vi "主副屏通信slave.vi"() -> ()   [LabVIEW 2016, in "斯坦道多参数.lvlib"]
uses:
  <vilib>/NI/Modbus Library/Network Protocol/Network Slave/TCP/Connection.ctl
  <vilib>/NI/Modbus Library/API/Wrapper/Create TCP Slave.vi
  <vilib>/NI/Modbus Library/API/slave/Modbus Slave.lvclass
  <vilib>/NI/Modbus Library/API/Wrapper/API Main.lvlib
  <vilib>/NI/Modbus Library/Network Protocol/Network Slave/TCP/TCP Slave.lvclass
panel:
  out "TCP Connection List":T1[](array[typedef])
  out "TCP Connection Count":u32
  in  "停止":bool
  out "read values":u16[](array[numeric])
  in  "write values":u16[](array[numeric])
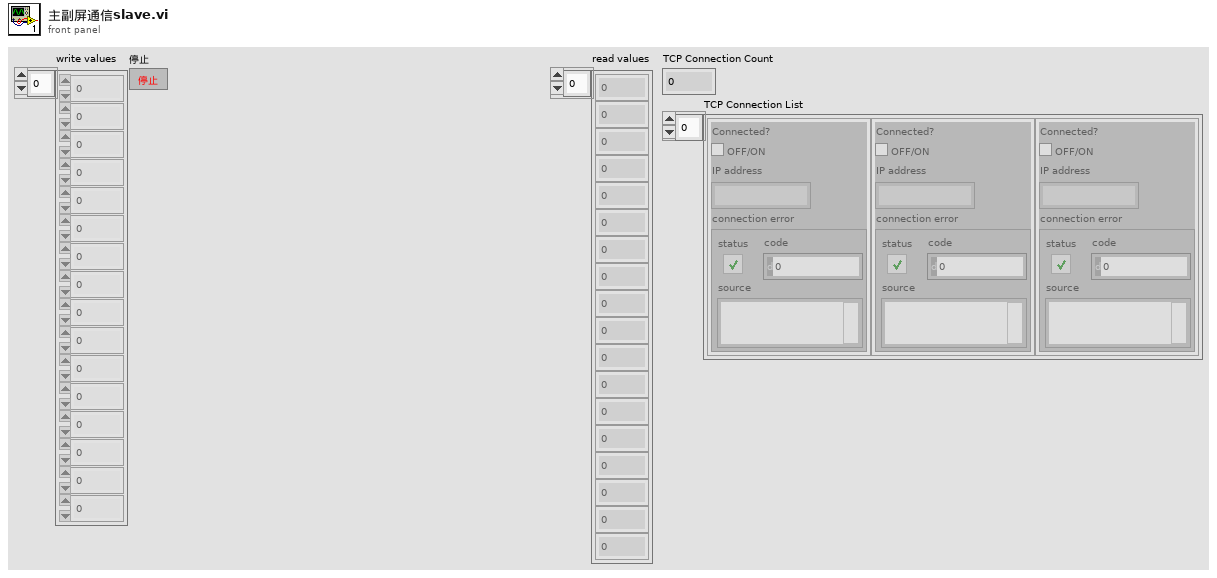
[diagram p1: front panel]
types:
  T1 = typedef "TCP Slave.lvclass/Connection.ctl" = cluster{"Connected?":bool, "IP address":string, "connection error":errorcluster}
  T2 = cluster{"数据保存间隔":dbl, "保存组数":dbl, "水温标样值":dbl, "pH标样值":dbl, "溶解氧标样值":dbl, "电导率标样值":dbl, "浊度标样值":dbl, "pH启用":bool, "溶解氧启用":bool, "电导率启用":bool, "浊度启用":bool}
  T3 = cluster{"数据保存间隔":dbl, "水温标样值":dbl, "pH标样值":dbl, "溶解氧标样值":dbl, "电导率标样值":dbl, "浊度标样值":dbl}
  T4 = cluster{"ph":bool, "DO":bool, "Cond":bool, "Turb":bool, "叶绿素a":bool, "藻密度":bool, "ORP":bool, "COD":bool}
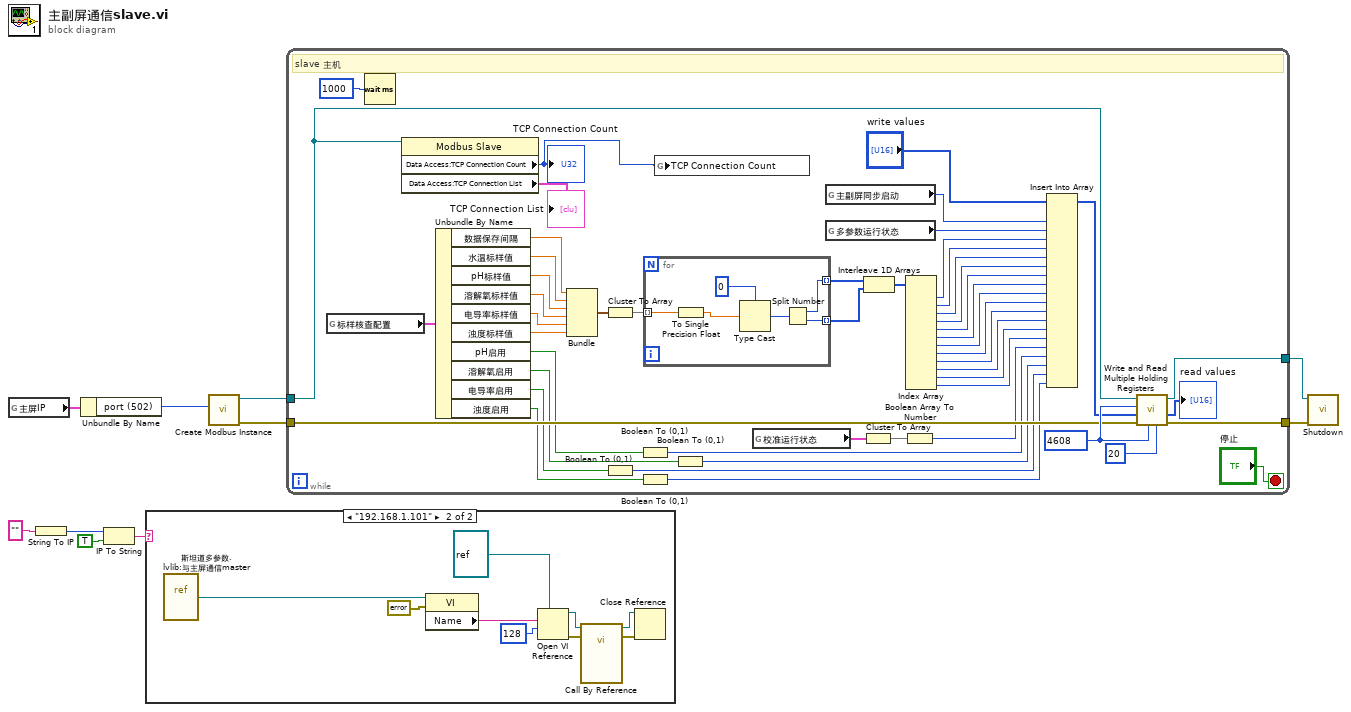
[diagram p0: block diagram]
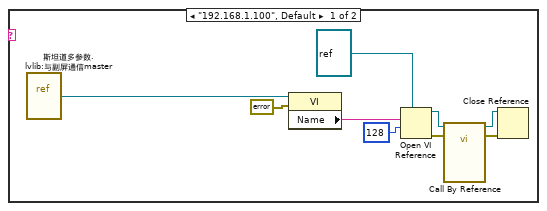
[diagram p2: hidden frame]
diagram:
  n1 = global read "多参数全局变量.vi" "主屏IP"() -> (w6:cluster{"address":string, "port (502)":u16})
  n2 = String To IP(1:"" ("名称")) -> (0:w4:u32)
  n3 = Unbundle By Name(w6) -> ("port (502)"=w5:u16)
  n4 = IP To String(1:TRUE ("句点符号？(F)"), 2:w4) -> (0:w1:string)
  n5 = case shown="\"192.168.1.101\"" w1 {
    frame "192.168.1.100", Default {
      n6 = vi-ref "斯坦道多参数.lvlib:与副屏通信master.vi"() -> (w11:refnum<vi>)
      n7 = property class="VI"(reference=w11, error in=errorcluster {"status"=FALSE, "code"=0, "source"=""} ("错误输出")) -> ("Name"=w12:string)  [unwired: 2 out]
      n8 = Open VI Reference(type specifier VI Refnum (for type only)=refnum<vi> refnum, vi path=w12, options=128 ("选项")) -> (vi reference=w14:refnum<vi>, error out=w16:errorcluster)  [unwired: 3 in]
      n9 = call-by-ref "?"(reference=w14, error in=w16) -> (reference out=w18:refnum<vi>, error out=w17:errorcluster)  [unwired: 12 in]
      n10 = Close Reference(reference=w18, error in (no error)=w17) -> ()  [unwired: 1 out]
    }
    frame "192.168.1.101" {
      n11 = vi-ref "斯坦道多参数.lvlib:与主屏通信master.vi"() -> (w20:refnum<vi>)
      n12 = property class="VI"(reference=w20, error in=errorcluster {"status"=FALSE, "code"=0, "source"=""} ("错误输出")) -> ("Name"=w21:string)  [unwired: 2 out]
      n13 = Open VI Reference(type specifier VI Refnum (for type only)=refnum<vi> refnum, vi path=w21, options=128 ("选项")) -> (vi reference=w23:refnum<vi>, error out=w25:errorcluster)  [unwired: 3 in]
      n14 = call-by-ref "?"(reference=w23, error in=w25) -> (reference out=w27:refnum<vi>, error out=w26:errorcluster)  [unwired: 12 in]
      n15 = Close Reference(reference=w27, error in (no error)=w26) -> ()  [unwired: 1 out]
    }
  }
  n16 = call-poly <vilib>:"Create Modbus Instance.vi"("port (502)"=w5) -> ("error out"=w7:errorcluster, "TCP slave instance"=w10:refnum<class "Modbus Slave.lvclass">)  [unwired: 9 in]
  n17 = while {
    tunnel: w10 -> [w31]
    tunnel: [w75] -> w9
    tunnel: [w74] -> w8
    tunnel: w7 -> [w73]
    stop <- "停止" stop-if-true
    w78 = u16 4608 ("write starting address")
    # "slave 主机"
    n18 = global read "断电保存变量.vi" "标样核查配置"() -> (w48:T2)
    n19 = Wait (ms)(milliseconds to wait=u32 1000 ("等待时间（毫秒）")) -> ()  [unwired: 1 out]
    n20 = property class="Modbus Slave"(reference=w31) -> ("Data Access:TCP Connection Count"=w29:u32, "Data Access:TCP Connection List"=→"TCP Connection List":T1[])  [unwired: 1 in, 2 out]
    "TCP Connection Count" <- w29
    n21 = Unbundle By Name(w48) -> ("数据保存间隔"=w47:dbl, "水温标样值"=w46:dbl, "pH标样值"=w45:dbl, "溶解氧标样值"=w44:dbl, "电导率标样值"=w43:dbl, "浊度标样值"=w42:dbl, "pH启用"=w40:bool, "溶解氧启用"=w37:bool, "电导率启用"=w38:bool, "浊度启用"=w39:bool)
    n22 = Bundle("数据保存间隔"=w47, "水温标样值"=w46, "pH标样值"=w45, "溶解氧标样值"=w44, "电导率标样值"=w43, "浊度标样值"=w42) -> (w41:T3)  [unwired: 1 in]
    n23 = Cluster To Array(cluster=w41) -> (array=w67:dbl[])
    n24 = Boolean To (0,1)(Boolean=w38) -> (0, 1=w34:i16)
    n25 = Boolean To (0,1)(Boolean=w40) -> (0, 1=w36:i16)
    n26 = Boolean To (0,1)(Boolean=w39) -> (0, 1=w33:i16)
    n27 = for {
      tunnel: w67 -> [w80] mode=indexing
      tunnel: [w82] -> w66 mode=indexing
      tunnel: [w81] -> w65 mode=indexing
      n28 = To Single Precision Float(number=w80) -> (single precision float=w79:sgl)
      n29 = Type Cast(type=0, x=w79) -> (*(type *) &x=w83:i32)
      n30 = Split Number(x=w83) -> (hi(x)=w82:u16, lo(x)=w81:u16)
    }
    n31 = global write "多参数全局变量.vi" "TCP Connection Count"(w29) -> ()
    n32 = Boolean To (0,1)(Boolean=w37) -> (0, 1=w35:i16)
    n33 = global read "多参数全局变量.vi" "校准运行状态"() -> (w51:T4)
    n34 = global read "多参数全局变量.vi" "主副屏同步启动"() -> (w69:u16)
    n35 = global read "多参数全局变量.vi" "多参数运行状态"() -> (w68:u16)
    n36 = Cluster To Array(cluster=w51) -> (array=w50:bool[])
    n37 = Interleave 1D Arrays(w66, w65) -> (w64:u16[])
    n38 = Boolean Array To Number(Boolean array=w50) -> (number=w49:u32)
    n39 = Index Array(array=w64) -> (element #1=w63:u16, element #2=w62:u16, element #3=w61:u16, element #4=w60:u16, element #5=w59:u16, element #6=w58:u16, element #7=w57:u16, element #8=w56:u16, element #9=w55:u16, element #10=w54:u16, element #11=w53:u16, element #12=w52:u16)  [unwired: 12 in]
    n40 = Insert Into Array(array="write values", new element #1=w69, new element #2=w68, new element #3=w63, new element #4=w62, new element #5=w61, new element #6=w60, new element #7=w59, new element #8=w58, new element #9=w57, new element #10=w56, new element #11=w55, new element #12=w54, new element #13=w53, new element #14=w52, new element #15=w49, new element #16=w36, new element #17=w35, new element #18=w34, new element #19=w33) -> (w32:u16[])  [unwired: 1 in]
    n41 = call-dynamic "Write and Read Multiple Holding Registers.vi"("read count"=u16 20, "read starting address"=w78, "error in"=w73, "write values"=w32, "write starting address"=w78, "Modbus instance in"=w31) -> ("error out"=w74:errorcluster, "read values"=→"read values":u16[], "Modbus instance out"=w75:refnum<class "Modbus Slave.lvclass">)  [unwired: 3 in]
  }
  n42 = call-dynamic "Shutdown.vi"("error in"=w8, "Modbus slave in"=w9) -> ()  [unwired: 9 in, 1 out]
